vi "get_item_type.vi"(8 "error in (no error)":errorcluster, 11 "Item in":refnum<class "Item.lvclass">) -> (0 "error out":errorcluster, 2 "item_type":T1, 3 "Item out":refnum<class "Item.lvclass">)   [LabVIEW 2020, in "toml_edit.lvlib" / "Item.lvclass"]
uses:
  Item.lvclass
  type--enum.ctl
  Item.lvclass/Item.ctl
  toml_edit.lvlib
  dragon_toml_64.dll
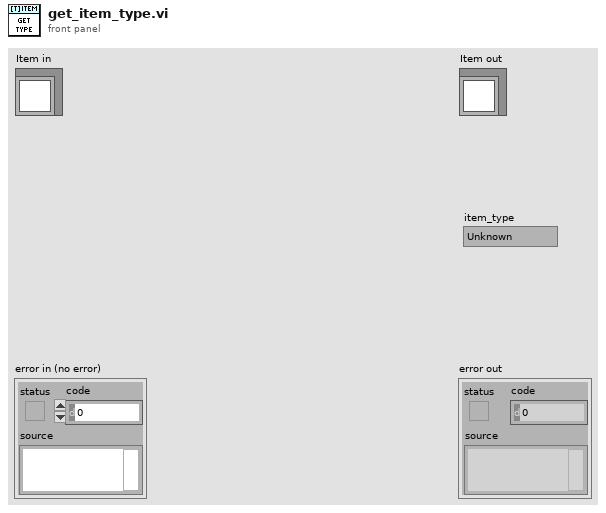
[diagram p1: front panel]
types:
  T1 = typedef "toml_edit.lvlib/Item.lvclass/type--enum.ctl" = enum16{"Unknown", "None", "Value", "ArrayOfTables", "Table"}
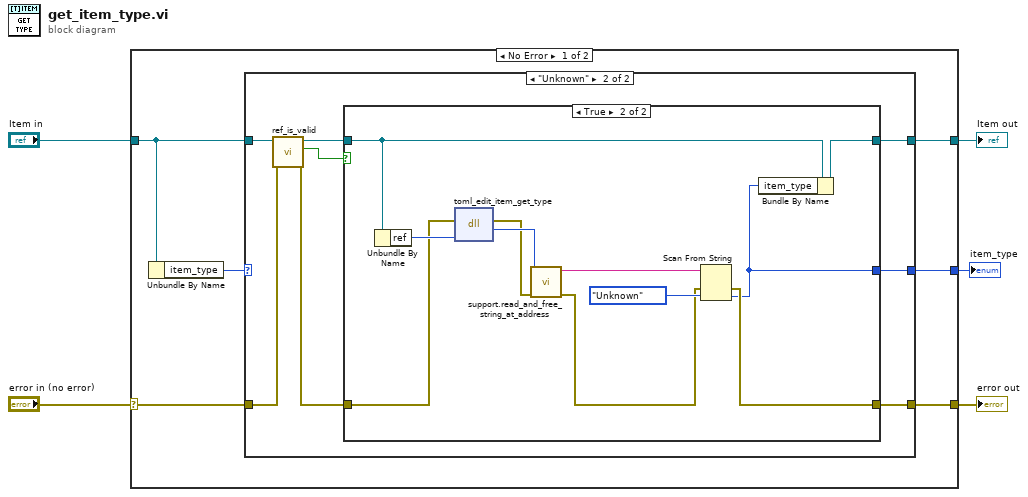
[diagram p0: block diagram]
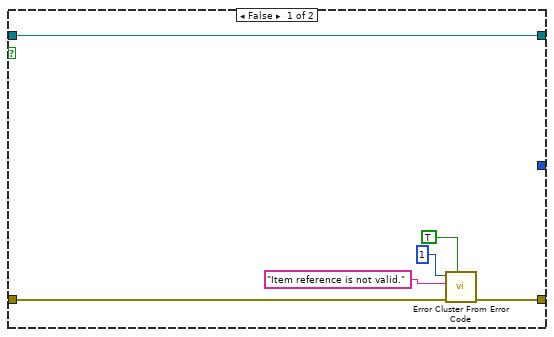
[diagram p3: hidden frame]
diagram:
  n1 = case shown="No Error" "error in (no error)" {
    selector: "error in (no error)" -> [w11 w41]
    tunnel: [w10 w41] -> w4
    tunnel: [w9 w40] -> w2
    tunnel: "Item in" -> [w7 w40]
    tunnel: [w8 _] -> w1
    frame No Error {
      n2 = Unbundle By Name(w7) -> ("item_type"=w6:T1)
      n3 = case shown="\"Unknown\"" w6 {
        selector: w6 -> [w13 _]
        tunnel: w11 -> [w12 w16]
        tunnel: [w12 w22] -> w10
        tunnel: [w14 w21] -> w9
        tunnel: [w13 w20] -> w8
        tunnel: w7 -> [w14 w18]
        frame Default {
        }
        frame "Unknown" {
          n4 = call-dynamic "ref_is_valid.vi"("error in (no error)"=w16, "Item in"=w18) -> ("error out"=w17:errorcluster, "ref_is_valid?"=w15:bool, "Item out"=w19:refnum<class "Item.lvclass">)  [unwired: 7 in]
          n5 = case shown="True" w15 {
            tunnel: [w28 w33] -> w22
            tunnel: [w23 w32] -> w21
            tunnel: [_ w31] -> w20
            tunnel: w19 -> [w23 w30]
            tunnel: w17 -> [w27 w29]
            frame False {
              n6 = call <vilib>:"Error Cluster From Error Code.vi"("show call chain? (False)"=TRUE, "error in (no error)"=w27, "error message (\"\")"="Item reference is not valid." ("error message (\"\")"), "error code (0)"=1) -> ("error out"=w28:errorcluster)  [unwired: 5 in]
            }
            frame True {
              n7 = Unbundle By Name(w30) -> ("ref"=w37:u64)
              n8 = dll-call lib="C:/Projects/labview-project-load-tools/source/submodules/toml-edit-labview/lv_src/dragon_toml_*.*" fn="toml_edit_item_get_type"(error in=w29, "item_ref"=w37) -> (error out=w38:errorcluster, "string_ptr"=w39:u64)  [unwired: 3 in, 1 out]
              n9 = call "support.read_and_free_string_at_address.vi"("error in (no error)"=w38, "string_ptr"=w39) -> ("error out"=w34:errorcluster, "string"=w35:string)  [unwired: 8 in]
              n10 = Scan From String(input string=w35, error in=w34, default 1=type--enum."Unknown" ("type")) -> (error out=w33:errorcluster, output 1=w31:T1)  [unwired: 2 in, 2 out]
              n11 = Bundle By Name(cluster=w30, "item_type"=w31) -> (w32:refnum<class "Item.lvclass">)
            }
          }
        }
      }
    }
    frame Error {
    }
  }
  "error out" <- w4
  "Item out" <- w2
  "item_type" <- w1
